vi "Set Address device.vi"(8 "error in (no error)":errorcluster caption="entrée d'erreur (pas d'erreur)", 10 "Device @":string, 11 "Class Instrument Multimeter en entrée":refnum<class "Class Instrument Balance.lvclass">) -> (0 "error out":errorcluster caption="sortie d'erreur", 3 "Class Instrument Multimeter en sortie":refnum<class "Class Instrument Balance.lvclass">)   [LabVIEW 2020, in "Library Instrument & Equipement.lvlib" / "Library Instruments.lvlib" / "Class Instrument Balance.lvclass"]
uses:
  Class Instrument Balance.lvclass
  Class Instrument Balance.lvclass/Class Instrument Balance.ctl
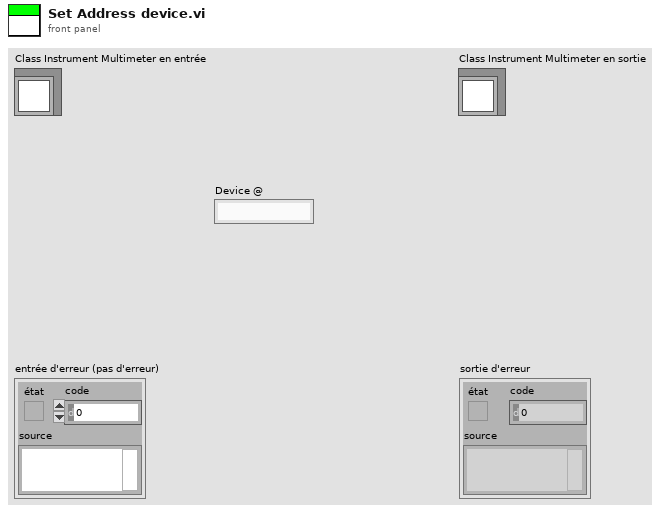
[diagram p1: front panel]
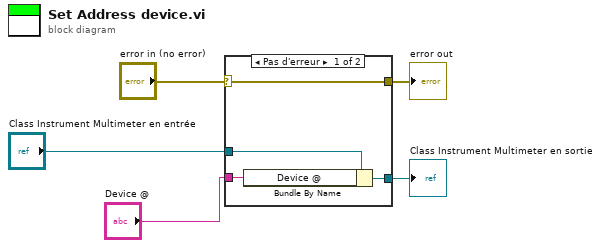
[diagram p0: block diagram]
diagram:
  n1 = case shown="Pas d'erreur" "error in (no error)" {
    selector: "error in (no error)" -> [w9 w11]
    tunnel: [w9 w11] -> w4
    tunnel: [w7 w10] -> w2
    tunnel: "Class Instrument Multimeter en entrée" -> [w8 w10]
    tunnel: "Device @" -> [w6 _]
    frame No Error {
      n2 = Bundle By Name(cluster=w8, "Device @"=w6) -> (w7:refnum<class "Class Instrument Balance.lvclass">)
    }
    frame Error {
    }
  }
  "error out" <- w4
  "Class Instrument Multimeter en sortie" <- w2
